vi "STEPRSLT.vi"(0 "VISA resource name":refnum<visa-resource-name>, 1 "Step Number":string, 2 "Amp or Ohm?":bool=TRUE, 7 "error in (no error)":errorcluster) -> (14 "Test Step Result":string="\r\n", 15 "Peak ARC Current (uA)":dbl, 16 "Execution Status":string, 17 "Measurement Result Unit":string, 18 "Elapsed Time (s)":dbl, 19 "Measurement Result (uA or mOhm)":dbl caption="Measurement Result(uA)", 20 "VISA resource name out":refnum<visa-resource-name>, 21 "Step Status":string, 22 "Final Test Level (A or V)":dbl, 23 "Peak Breakdown Current (uA)":dbl caption="Peak Breakdown Current(uA)", 24 "Peak Breakdown Current Unit":string, 25 "Error Message":string, 26 "Error Code":i32, 27 "error out":errorcluster)   [LabVIEW 2010, in "VITREK V7X.lvlib"]
doc: "Responds with a set of fields giving the complete set of results for the speciified test step.\n\n<b>Note:</b> please refer to the instrument manual for the <b>STEPSLT?, <NR1></b> specification."
uses:
  VITREK V7X.lvlib
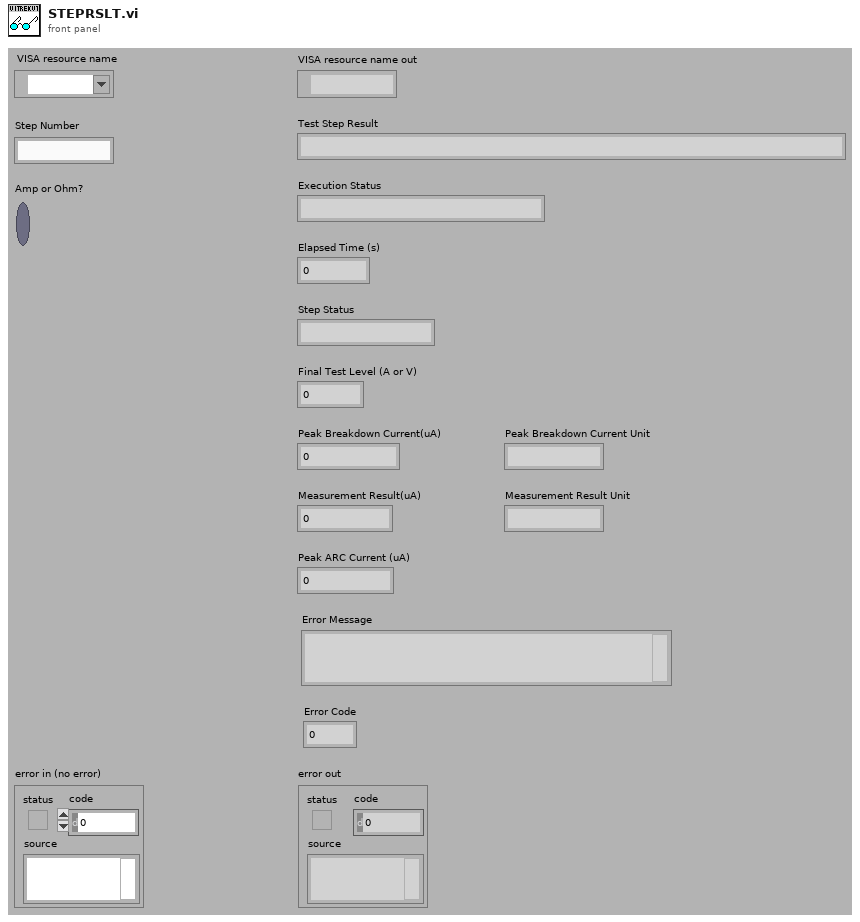
[diagram p1: front panel]
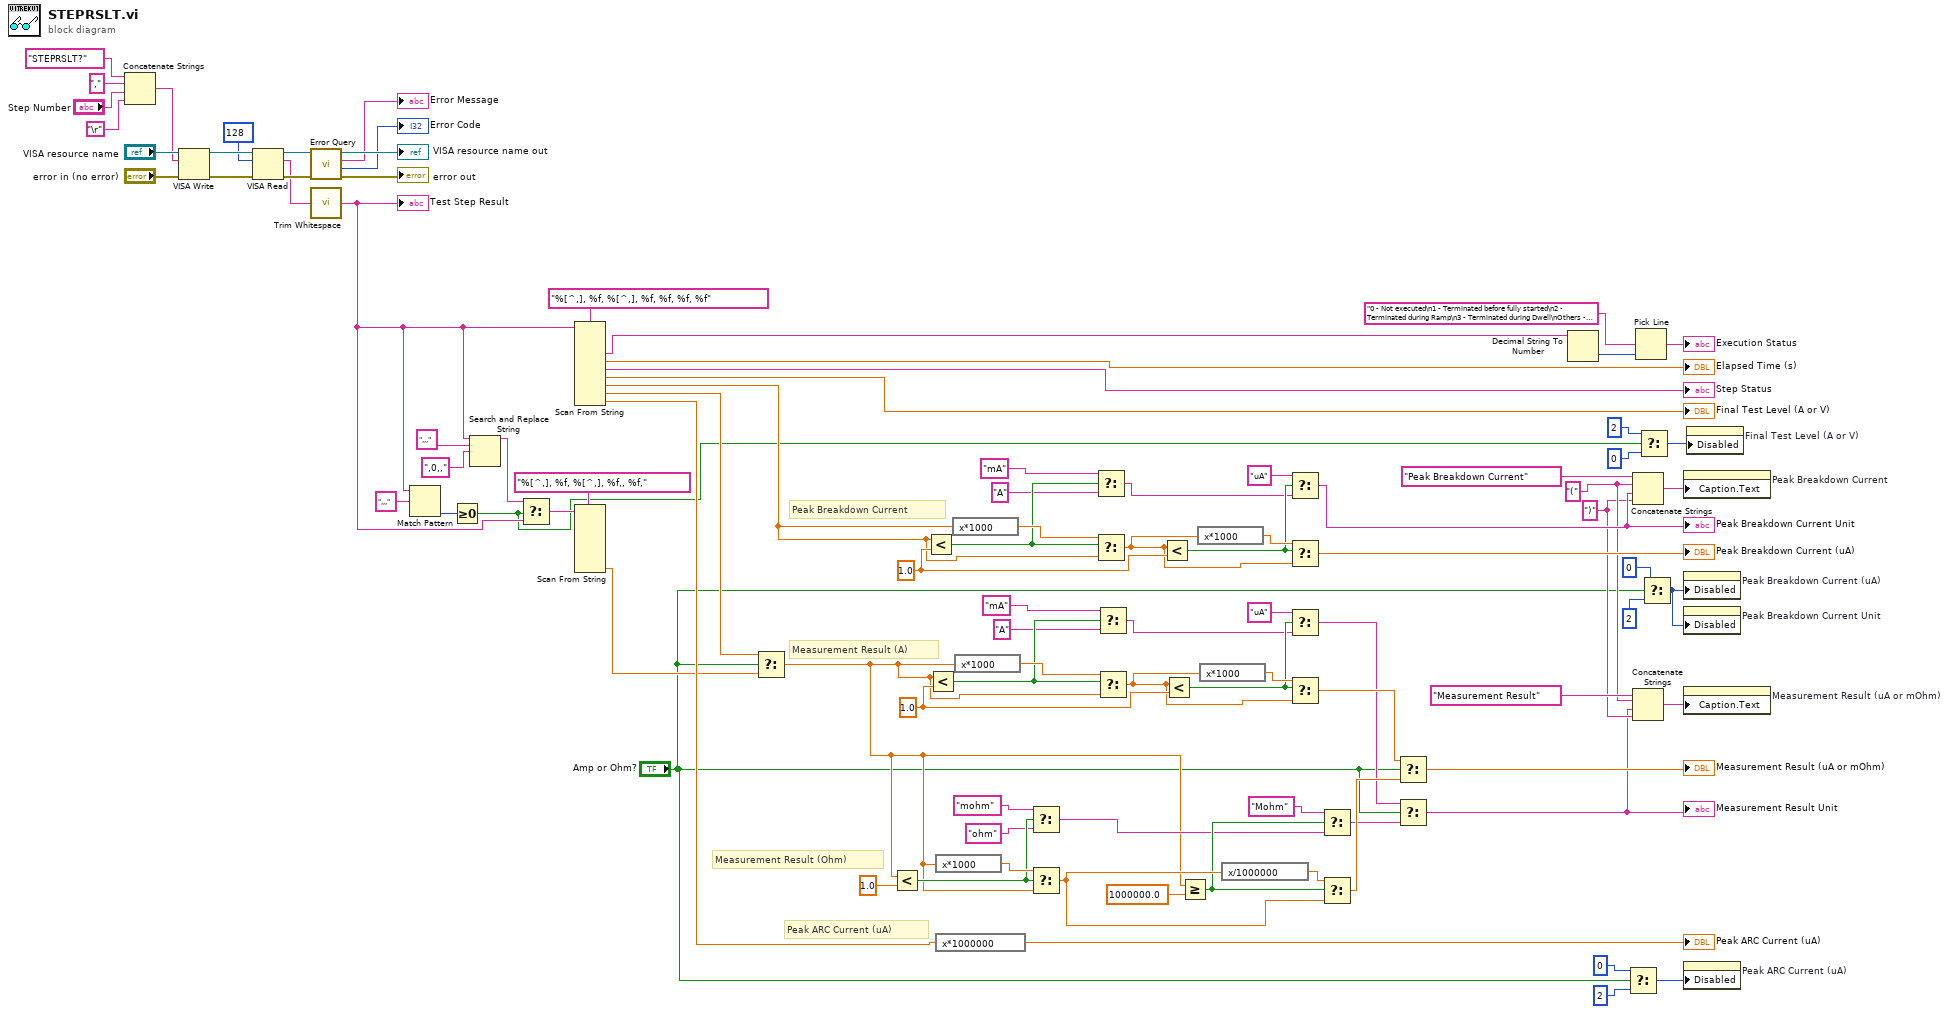
[diagram p0: block diagram]
diagram:
  w51 = 1.0 ("y")
  w37 = ")"
  w38 = "("
  w77 = 1.0 ("y")
  # "Peak ARC Current (uA)"
  # "Measurement Result (Ohm)"
  # "Measurement Result (A)"
  # "Peak Breakdown Current"
  n1 = Concatenate Strings("STEPRSLT?", ",", "Step Number", "\r") -> (w84:string)
  n2 = VISA Write(VISA resource name="VISA resource name", write buffer=w84, error in (no error)="error in (no error)") -> (VISA resource name out=w91:refnum<visa-resource-name>, error out=w89:errorcluster)  [unwired: 1 out]
  n3 = VISA Read(VISA resource name=w91, byte count=u32 128, error in (no error)=w89) -> (VISA resource name out=w90:refnum<visa-resource-name>, read buffer=w86:string, error out=w87:errorcluster)  [unwired: 1 out]
  n4 = call "Error Query.vi"("error in (no error)"=w87, "VISA resource name"=w90) -> ("error out"=→"error out":errorcluster, "Error Code"=→"Error Code":i32, "Error Message"=→"Error Message":string, "VISA resource name out"=→"VISA resource name out":refnum<visa-resource-name>)  [unwired: 6 in]
  n5 = call <vilib>:"Trim Whitespace.vi"("string"=w86) -> ("trimmed string"=w18:string)  [unwired: 1 in]
  "Test Step Result" <- w18
  n6 = Match Pattern(string=w18, regular expression=",,,") -> (offset past match=w22:i32)  [unwired: 1 in, 3 out]
  n7 = Greater Or Equal To 0?(x=w22) -> (x >= 0?=w9:bool)
  n8 = Search and Replace String(input string=w18, search string=",,,", replace string=",0,,") -> (result string=w19:string)  [unwired: 5 in, 3 out]
  n9 = Select(t=w19, s=w9, f=w18) -> (s? t:f=w17:string)
  n10 = Scan From String(format string="%[^,], %f, %[^,], %f, %f, %f, %f", input string=w18) -> (output 1=w3:string, output 2=→"Elapsed Time (s)":dbl, output 3=→"Step Status":string, output 4=→"Final Test Level (A or V)":dbl, output 5=w26:dbl, output 6=w27:dbl, output 7=w25:dbl)  [unwired: 9 in, 3 out]
  n11 = Scan From String(format string="%[^,], %f, %[^,], %f,, %f,", input string=w17) -> (output 5=w24:dbl)  [unwired: 11 in, 3 out]
  n12 = Select(t=w27, s="Amp or Ohm?", f=w24) -> (s? t:f=w28:dbl)
  n13 = Less?(x=w28, y=1.0) -> (x < y?=w59:bool)
  n14 = Less?(x=w26, y=w77) -> (x < y?=w73:bool)
  n15 = Less?(x=w28, y=w51) -> (x < y?=w47:bool)
  n16 = expression code="x*1000"(w28) -> (w62:dbl)
  n17 = expression code="x*1000000"(w25) -> (→"Peak ARC Current (uA)":dbl)
  n18 = expression code="x*1000"(w26) -> (w75:dbl)
  n19 = expression code="x*1000"(w28) -> (w49:dbl)
  n20 = Select(t="mohm", s=w59, f="ohm") -> (s? t:f=w54:string)
  n21 = Select(t=w62, s=w59, f=w28) -> (s? t:f=w60:dbl)
  n22 = Select(t="mA", s=w73, f="A") -> (s? t:f=w69:string)
  n23 = Select(t=w75, s=w73, f=w26) -> (s? t:f=w76:dbl)
  n24 = Select(t="mA", s=w47, f="A") -> (s? t:f=w43:string)
  n25 = Select(t=w49, s=w47, f=w28) -> (s? t:f=w50:dbl)
  n26 = Less?(x=w76, y=w77) -> (x < y?=w71:bool)
  n27 = Less?(x=w50, y=w51) -> (x < y?=w45:bool)
  n28 = Greater Or Equal?(x=w28, y=1000000.0) -> (x >= y?=w56:bool)
  n29 = expression code="x*1000"(w76) -> (w78:dbl)
  n30 = expression code="x*1000"(w50) -> (w52:dbl)
  n31 = expression code="x/1000000"(w60) -> (w61:dbl)
  n32 = Select(t="uA", s=w71, f=w69) -> (s? t:f=w65:string)
  "Peak Breakdown Current Unit" <- w65
  n33 = Select(t=w78, s=w71, f=w76) -> (s? t:f=→"Peak Breakdown Current (uA)":dbl)
  n34 = Select(t="uA", s=w45, f=w43) -> (s? t:f=w41:string)
  n35 = Select(t=w52, s=w45, f=w50) -> (s? t:f=w42:dbl)
  n36 = Select(t="Mohm", s=w56, f=w54) -> (s? t:f=w40:string)
  n37 = Select(t=w61, s=w56, f=w60) -> (s? t:f=w53:dbl)
  n38 = Select(t=w42, s="Amp or Ohm?", f=w53) -> (s? t:f=→"Measurement Result (uA or mOhm)":dbl)
  n39 = Select(t=w41, s="Amp or Ohm?", f=w40) -> (s? t:f=w35:string)
  "Measurement Result Unit" <- w35
  n40 = Decimal String To Number(string=w3) -> (number=w4:i32)  [unwired: 2 in, 1 out]
  n41 = Select(t=0, s="Amp or Ohm?", f=2) -> (s? t:f=w16:i32)
  n42 = Concatenate Strings("Peak Breakdown Current", w38, w65, w37) -> (w66:string)
  n43 = Concatenate Strings("Measurement Result", w38, w35, w37) -> (w36:string)
  n44 = Pick Line(multi-line string="0 - Not executed\n1 - Terminated before fully started\n2 - Terminated during Ramp\n3 - Terminated during Dwell\nOthers - Terminated", line index=w4) -> (output string=→"Execution Status":string)  [unwired: 1 in]
  n45 = Select(t=2, s=w9, f=0) -> (s? t:f=w10:i32)
  n46 = Select(t=0, s="Amp or Ohm?", f=2) -> (s? t:f=w6:i32)
  n47 = property on="Peak Breakdown Current" class="DigNum (strict)"("Caption.Text"=w66) -> ()  [unwired: 2 in, 2 out]
  n48 = property on="Peak Breakdown Current (uA)" class="DigNum (strict)"("Disabled"=w6) -> ()  [unwired: 2 in, 2 out]
  n49 = property on="Peak Breakdown Current Unit" class="Str"("Disabled"=w6) -> ()  [unwired: 2 in, 2 out]
  n50 = property on="Measurement Result (uA or mOhm)" class="DigNum (strict)"("Caption.Text"=w36) -> ()  [unwired: 2 in, 2 out]
  n51 = property on="Peak ARC Current (uA)" class="DigNum (strict)"("Disabled"=w16) -> ()  [unwired: 2 in, 2 out]
  n52 = property on="Final Test Level (A or V)" class="DigNum (strict)"("Disabled"=w10) -> ()  [unwired: 2 in, 2 out]
